vi "RecCOMsg.vi"(9 "tsapp_receive_can_messageList":T1[](array[typedef])) -> (0 "CORecSDOData":u32 caption="接收数据" format="0x%04x", 1 "接收子索引":u8=1, 2 "接收索引":u16 caption="索引" format="0x%04x", 3 "接收从站号":u8 caption="从站号" max=127, 4 "接收到的原始报文：":string)   [LabVIEW 2016]
uses:
  MessageInfo.ctl
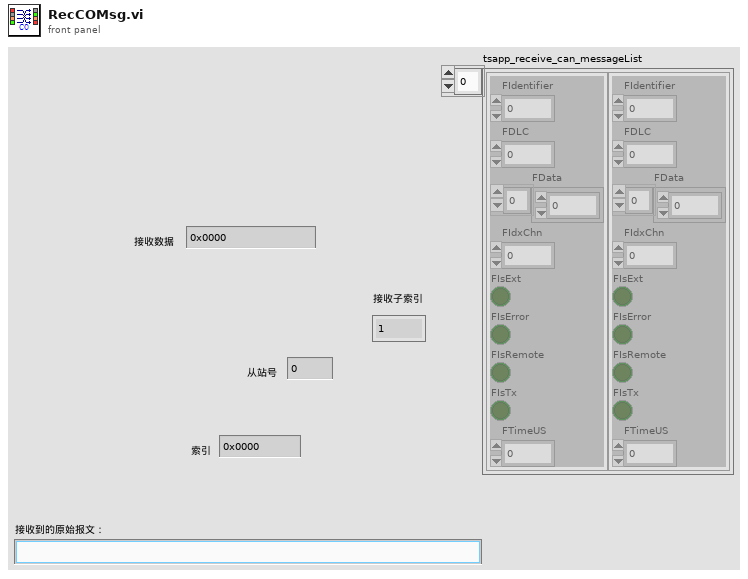
[diagram p1: front panel]
types:
  T1 = typedef "MessageInfo.ctl" = cluster{"FIdentifier":i32, "FDLC":u8, "FData":u8[], "FIdxChn":u8, "FIsExt":bool, "FIsError":bool, "FIsRemote":bool, "FIsTx":bool, "FTimeUS":u64}
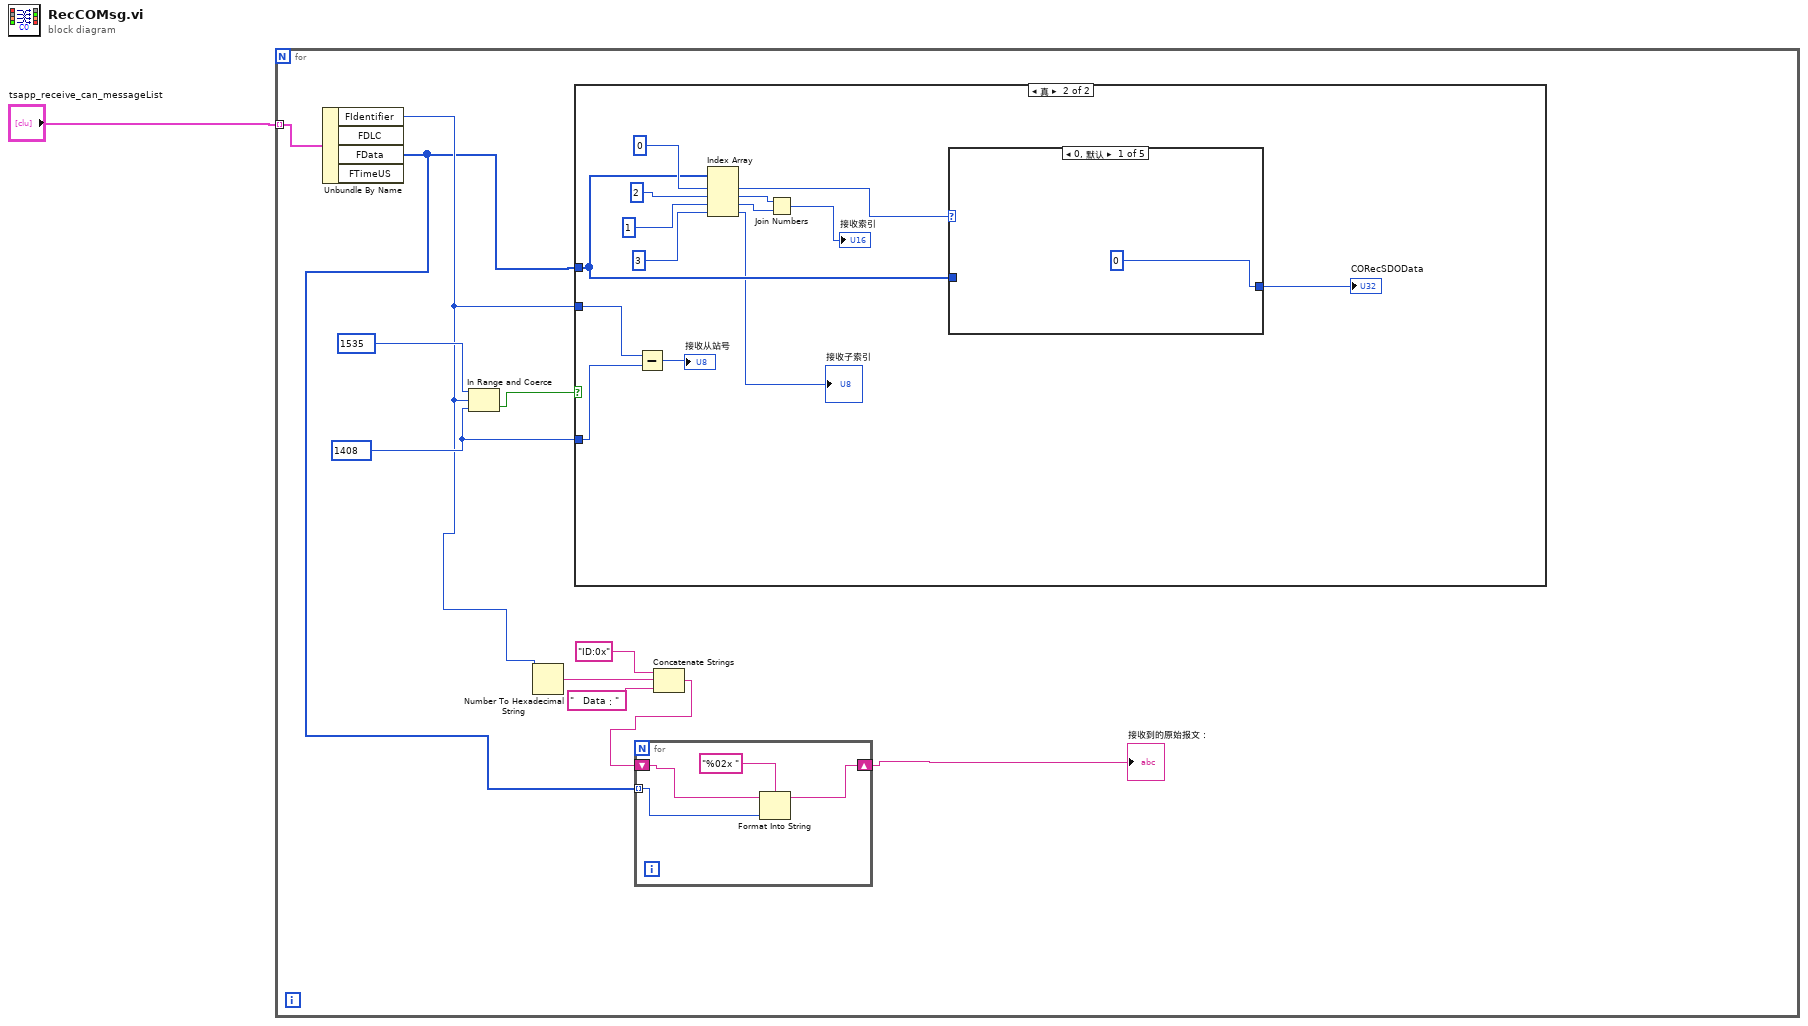
[diagram p0: block diagram]
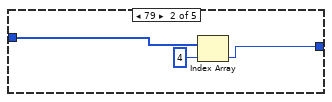
[diagram p3: hidden frame]
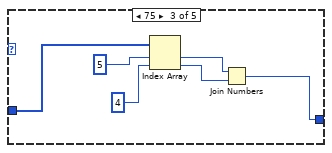
[diagram p4: hidden frame]
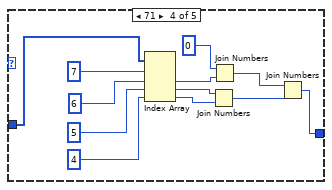
[diagram p5: hidden frame]
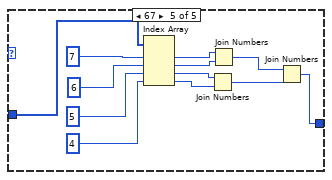
[diagram p6: hidden frame]
diagram:
  n1 = for {
    tunnel: "tsapp_receive_can_messageList" -> [w12] mode=indexing
    w9 = u32 1408 ("上限")
    n2 = Unbundle By Name(w12) -> ("FIdentifier"=w3:i32, "FData"=w2:u8[])  [unwired: 2 out]
    n3 = In Range and Coerce(upper limit=u32 1535 ("上限"), x=w3, lower limit=w9) -> (In Range?=w10:bool)  [unwired: 1 out]
    n4 = Number To Hexadecimal String(2:w3) -> (0:w7:string)  [unwired: 1 in]
    n5 = case shown="真" w10 {
      tunnel: w2 -> [_ w22]
      tunnel: w3 -> [_ w28]
      tunnel: w9 -> [_ w30]
      frame False {
      }
      frame True {
        n6 = Subtract(x=w28, y=w30) -> (x-y=→"接收从站号":u32)
        n7 = Index Array(array=w22, index #1=0 ("索引"), index #2=2 ("索引"), index #3=1 ("索引"), index #4=3 ("索引")) -> (element #1=w23:u8, element #2=w20:u8, element #3=w19:u8, element #4=→"接收子索引":u8)
        n8 = Join Numbers(hi=w20, lo=w19) -> ((hi.lo)=→"接收索引":u16)
        n9 = case shown="0, 默认" w23 {
          tunnel: w22 -> [_ w34 w40 w44 w54]
          tunnel: [u32 0 w32 w35 w41 w53] -> w21
          frame 0, Default {
          }
          frame 79 {
            n10 = Index Array(array=w34, index=4 ("索引")) -> (element=w32:u8)
          }
          frame 75 {
            n11 = Index Array(array=w40, index #1=5 ("索引"), index #2=4 ("索引")) -> (element #1=w37:u8, element #2=w36:u8)
            n12 = Join Numbers(hi=w37, lo=w36) -> ((hi.lo)=w35:u16)
          }
          frame 71 {
            n13 = Index Array(array=w44, index #1=7 ("索引"), index #2=6 ("索引"), index #3=5 ("索引"), index #4=4 ("索引")) -> (element #2=w48:u8, element #3=w49:u8, element #4=w50:u8)  [unwired: 1 out]
            n14 = Join Numbers(hi=w49, lo=w50) -> ((hi.lo)=w52:u16)
            n15 = Join Numbers(hi=u8 0, lo=w48) -> ((hi.lo)=w51:u16)
            n16 = Join Numbers(hi=w51, lo=w52) -> ((hi.lo)=w41:u32)
          }
          frame 67 {
            n17 = Index Array(array=w54, index #1=7 ("索引"), index #2=6 ("索引"), index #3=5 ("索引"), index #4=4 ("索引")) -> (element #1=w59:u8, element #2=w60:u8, element #3=w61:u8, element #4=w62:u8)
            n18 = Join Numbers(hi=w61, lo=w62) -> ((hi.lo)=w64:u16)
            n19 = Join Numbers(hi=w59, lo=w60) -> ((hi.lo)=w63:u16)
            n20 = Join Numbers(hi=w63, lo=w64) -> ((hi.lo)=w53:u32)
          }
        }
        "CORecSDOData" <- w21
      }
    }
    n21 = Concatenate Strings("ID:0x" ("字符串"), w7, "   Data：" ("字符串")) -> (w5:string)
    n22 = for {
      tunnel: w2 -> [w15] mode=indexing
      shift-right: [w14] -> w4
      shift-left: w5 -> [w13]
      n23 = Format Into String(format string="%02x " ("格式字符串"), initial string=w13, w15) -> (resulting string=w14:string)  [unwired: 1 in, 1 out]
    }
    "接收到的原始报文：" <- w4
  }
